vi "Throw Invalid JSON Error.vi"(7 "error source vi name":string, 8 "error in (no error)":errorcluster, 11 "name":string) -> (0 "error out":errorcluster)   [LabVIEW 2019, in "DSF Core.lvlib" / "Configuration Session.lvclass"]
uses:
  Configuration Session.lvclass
  Errors.ctl
  <vilib>/NI/Memory Manager/Static Errors.lvlib
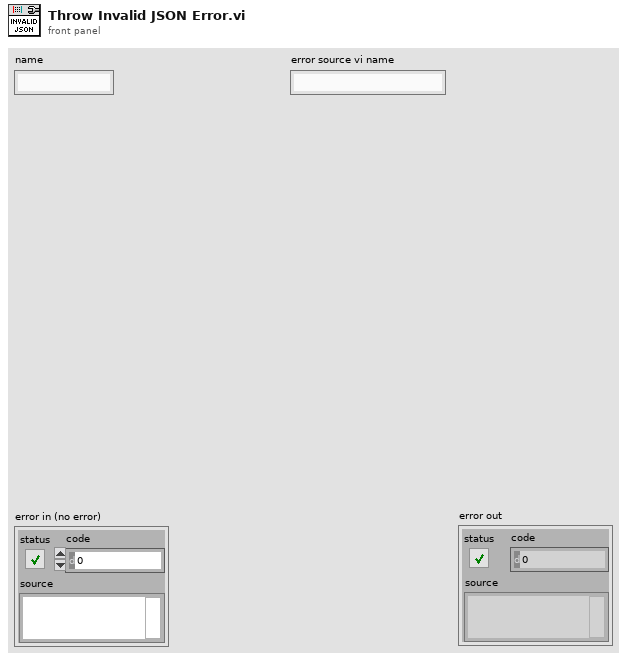
[diagram p1: front panel]
types:
  T1 = typedef "DSF Core.lvlib/Configuration Session.lvclass/Errors.ctl" = enum16{"Channel Overlap", "Invalid Engine Offset", "Invalid JSON"}
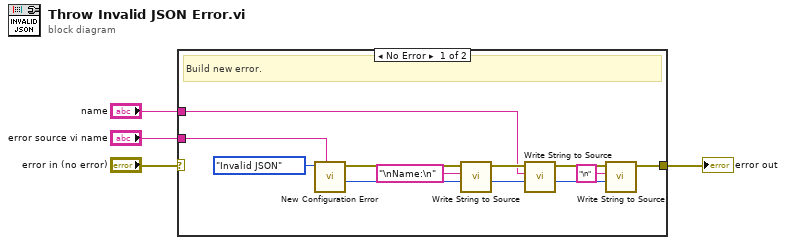
[diagram p0: block diagram]
diagram:
  n1 = case shown="No Error" "error in (no error)" {
    selector: "error in (no error)" -> [_ w17]
    tunnel: [w9 w17] -> w3
    tunnel: "error source vi name" -> [w11 _]
    tunnel: "name" -> [w8 _]
    frame No Error {
      # "Build new error."
      n2 = call "New Configuration Error.vi"("error source vi name"=w11, "configuration error"=Errors."Invalid JSON") -> ("new offset"=w15:i32, "error out"=w16:errorcluster)  [unwired: 8 in]
      n3 = call <vilib>:"Write String to Source.vi"("offset"=w15, "string"="\nName:\n", "error in"=w16) -> ("new offset"=w13:i32, "error out"=w14:errorcluster)  [unwired: 7 in]
      n4 = call <vilib>:"Write String to Source.vi"("offset"=w13, "string"=w8, "error in"=w14) -> ("new offset"=w12:i32, "error out"=w6:errorcluster)  [unwired: 7 in]
      n5 = call <vilib>:"Write String to Source.vi"("offset"=w12, "string"="\n", "error in"=w6) -> ("error out"=w9:errorcluster)  [unwired: 7 in, 1 out]
    }
    frame Error {
      # "Incoming error. Pass through."
    }
  }
  "error out" <- w3
